vi "Climb Joystick.vi"(2 "Operator D-Pad":i16) -> (0 "Climb Teleop Command":T1)   [LabVIEW 2019]
uses:
  Climb Command Type Def.ctl
  Climb Mode Type Def.ctl
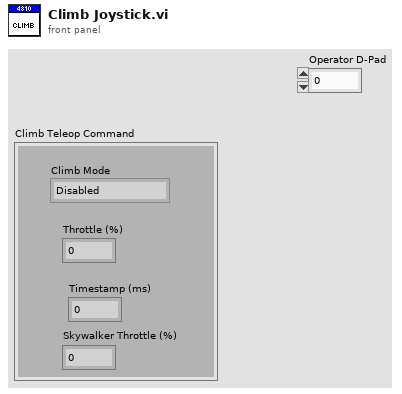
[diagram p1: front panel]
types:
  T1 = typedef "Climb Command Type Def.ctl" = cluster{"Climb Mode":T2, "Throttle (%)":dbl, "Timestamp (ms)":dbl, "Skywalker Throttle (%)":dbl}
  T2 = typedef "Climb Mode Type Def.ctl" = enum16{"Disabled", "Raw Throttle"}
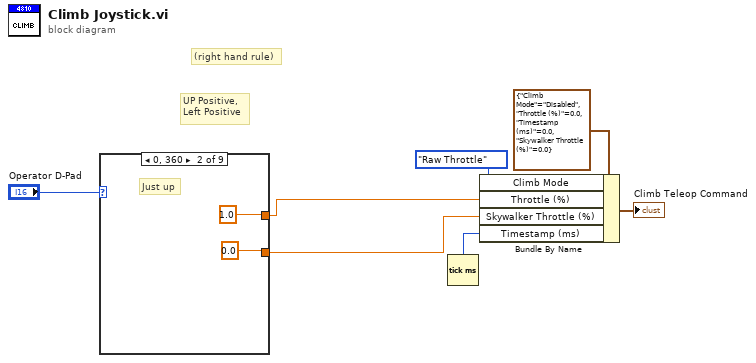
[diagram p0: block diagram]
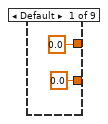
[diagram p2: hidden frame]
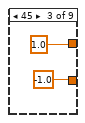
[diagram p3: hidden frame]
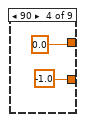
[diagram p4: hidden frame]
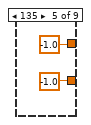
[diagram p5: hidden frame]
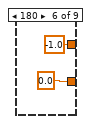
[diagram p6: hidden frame]
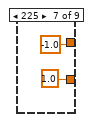
[diagram p7: hidden frame]
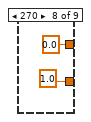
[diagram p8: hidden frame]
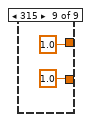
[diagram p9: hidden frame]
diagram:
  # "(right hand rule)"
  # "UP Positive, \nLeft Positive"
  n1 = case shown="0, 360" "Operator D-Pad" {
    tunnel: [0.0 1.0 1.0 0.0 -1.0 -1.0 -1.0 0.0 1.0] -> w2
    tunnel: [0.0 0.0 -1.0 -1.0 -1.0 0.0 1.0 1.0 1.0] -> w1
    frame Default {
    }
    frame 0, 360 {
      # "Just up"
    }
    frame 45 {
    }
    frame 90 {
    }
    frame 135 {
    }
    frame 180 {
    }
    frame 225 {
    }
    frame 270 {
    }
    frame 315 {
    }
  }
  n2 = Tick Count (ms)() -> (millisecond timer value=w4:u32)
  n3 = Bundle By Name(cluster=T1 {"Climb Mode"=enum."Disabled", "Throttle (%)"=0.0, "Timestamp (ms)"=0.0, "Skywalker Throttle (%)"=0.0} ("Climb Command"), "Climb Mode"=Climb_Mode_Type_Def."Raw Throttle", "Throttle (%)"=w2, "Skywalker Throttle (%)"=w1, "Timestamp (ms)"=w4) -> (→"Climb Teleop Command":T1)
